vi "lv error handling.vi"(8 "error in":errorcluster, 10 "error handle":i32, 11 "return code":i32) -> (0 "error out":errorcluster)   [LabVIEW 2026]
uses:
  bin/nominalClient_64.dll
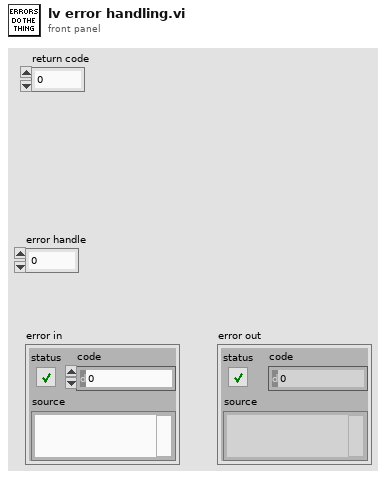
[diagram p1: front panel]
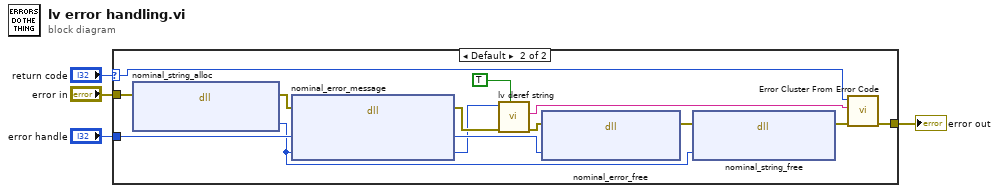
[diagram p0: block diagram]
diagram:
  n1 = case shown="Default" "return code" {
    selector: "return code" -> [_ w16]
    tunnel: "error in" -> [w5 w7]
    tunnel: [w5 w17] -> w4
    tunnel: "error handle" -> [_ w19]
    frame 0 {
    }
    frame Default {
      n2 = dll-call lib="C:/sw/nominal-c/bin/nominalClient_64.dll" fn="nominal_string_alloc"(error in=w7) -> (error out=w8:errorcluster, "string handle"=w6:i32)  [unwired: 4 in, 1 out]
      n3 = dll-call lib="C:/sw/nominal-c/bin/nominalClient_64.dll" fn="nominal_error_message"(error in=w8, "error handle"=w19, "string handle"=w6) -> (error out=w15:errorcluster, "error handle"=w18:i32, "string handle"=w13:i32)  [unwired: 3 in, 1 out]
      n4 = call "lv deref string.vi"("do not free"=TRUE, "error in"=w15, "string handle"=w13) -> ("error out"=w14:errorcluster, "outbuffer"=w11:string)  [unwired: 7 in]
      n5 = dll-call lib="C:/sw/nominal-c/bin/nominalClient_64.dll" fn="nominal_error_free"(error in=w14, "error handle"=w18) -> (error out=w10:errorcluster)  [unwired: 4 in, 1 out]
      n6 = dll-call lib="C:/sw/nominal-c/bin/nominalClient_64.dll" fn="nominal_string_free"(error in=w10, "string handle"=w6) -> (error out=w9:errorcluster)  [unwired: 4 in, 1 out]
      n7 = call <vilib>:"Error Cluster From Error Code.vi"("error in (no error)"=w9, "error message (\"\")"=w11, "error code (0)"=w16) -> ("error out"=w17:errorcluster)  [unwired: 6 in]
    }
  }
  "error out" <- w4
